vi "sppf single step.vi"(6 "do update":bool, 7 "dt":dbl, 8 "num green photons":dbl, 9 "num red photons":dbl, 10 "w":dbl[][](array[numeric])=[[1e-09, 0.0], [0.0, 1e-09]], 11 "theta":dbl[](array[numeric])=[0.0, 0.0]) -> (1 "wjjm1":dbl[][](array[numeric]), 2 "w":dbl[][](array[numeric]), 3 "theta":dbl[](array[numeric]))   [LabVIEW 2010]
uses:
  <vilib>/Analysis/baseanly.llb/Matrix Type of Inverse Matrix.ctl
  <vilib>/Analysis/Matrix/Datatypes/RealMatrix.ctl
  <vilib>/Analysis/Matrix/Numeric/Multiply/Multiply - R,RM.vi
  <vilib>/Analysis/Matrix/Numeric/Add/Add - RM,RM.vi
  <vilib>/Analysis/baseanly.llb/Real Inverse Matrix.vi
  <vilib>/Analysis/BLAS.llb/dgemv - General Matrix-Vector Product (DBL).vi
  <vilib>/Analysis/Matrix/NI_Matrix.lvlib
  <vilib>/Analysis/NI_AALBase.lvlib
  <vilib>/Analysis/NI_AALBLAS.lvlib
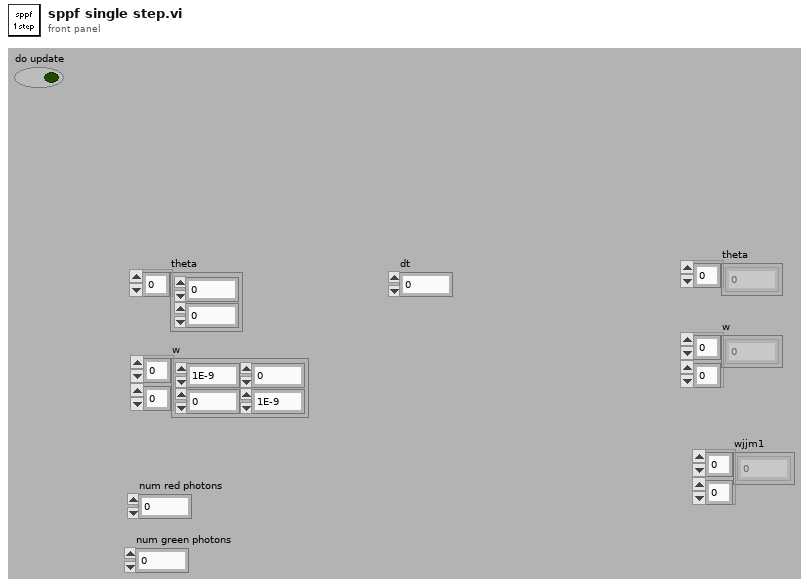
[diagram p1: front panel]
types:
  T1 = typedef "NI_Matrix.lvlib/RealMatrix.ctl" = dbl[][]
  T2 = typedef "NI_AALBase.lvlib/Matrix Type of Inverse Matrix.ctl" = enum32{"General", "Positive Definite", "Lower Triangular", "Upper Triangular"}
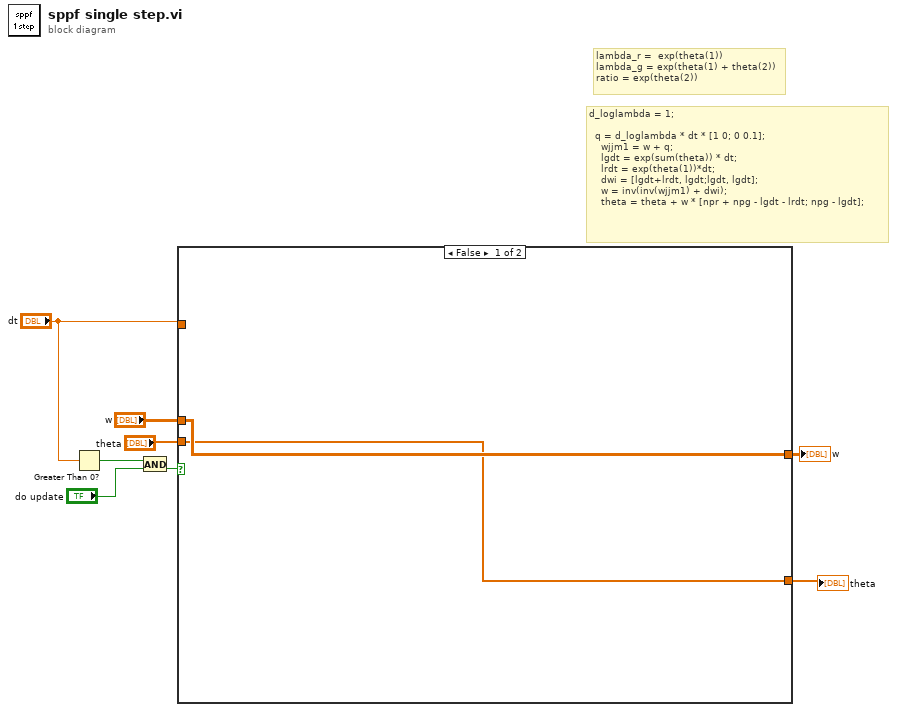
[diagram p0: block diagram]
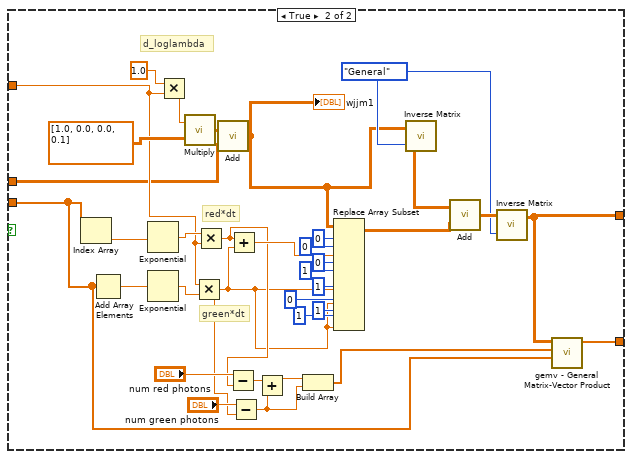
[diagram p2: hidden frame]
diagram:
  # "d_loglambda = 1;\n  \n  q = d_loglambda * dt * [1 0; 0 0.1];\n    wjjm1 = w + q;\n    lgdt = exp(sum(theta)) * dt;\n    lrdt = exp(theta(1))*dt;\n    dwi = [lgdt+lrdt, lgdt;lgdt, lgdt];\n    w = inv(inv(wjjm1) + dwi);\n    theta = theta + w * [npr + npg - lgdt - lrdt; npg - lgdt];"
  # "lambda_r =  exp(theta(1))\nlambda_g = exp(theta(1) + theta(2))\nratio = exp(theta(2))"
  n1 = Greater Than 0?(x="dt") -> (x > 0?=w2:bool)
  n2 = And(x=w2, y="do update") -> (x .and. y?=w3:bool)
  n3 = case shown="False" w3 {
    tunnel: "dt" -> [_ w39]
    tunnel: "theta" -> [w9 w17]
    tunnel: [w10 w16] -> w7
    tunnel: "w" -> [w10 w15]
    tunnel: [w9 w14] -> w5
    frame False {
    }
    frame True {
      w26 = Matrix_Type_of_Inverse_Matrix."General" ("matrix type")
      # "d_loglambda"
      # "green*dt"
      # "red*dt"
      n4 = Index Array(array=w17) -> (element=w43:dbl)  [unwired: 1 in]
      n5 = Add Array Elements(numeric array=w17) -> (sum=w42:dbl)
      n6 = Exponential(1:w43) -> (0:w41:dbl)
      n7 = Exponential(1:w42) -> (0:w40:dbl)
      n8 = Multiply(x=1.0, y=w39) -> (x*y=w13:dbl)
      n9 = call-poly <vilib>:"Multiply.vi"("Real Matrix A"=T1 [[1.0, 0.0], [0.0, 0.1]] ("Real Matrix"), "Real Scalar c"=w13) -> ("c * A"=w44:T1)
      n10 = Multiply(x=w39, y=w40) -> (x*y=w22:dbl)
      n11 = Multiply(x=w41, y=w39) -> (x*y=w24:dbl)
      n12 = call-poly <vilib>:"Add.vi"("Real Matrix B"=w15, "Real Matrix A"=w44) -> ("A + B"=w11:T1)
      "wjjm1" <- w11
      n13 = Subtract(x="num red photons", y=w24) -> (x-y=w21:dbl)
      n14 = Add(x=w24, y=w22) -> (x+y=w30:dbl)
      n15 = Subtract(x="num green photons", y=w22) -> (x-y=w19:dbl)
      n16 = Add(x=w21, y=w19) -> (x+y=w20:dbl)
      n17 = Build Array(w20, w19) -> (w18:dbl[])
      n18 = Replace Array Subset(array=w11, new element #1=w30, index (row) #1=0 ("disabled index (row)"), index (col) #1=0 ("disabled index (col)"), new element #2=w22, index (row) #2=0 ("index (row)"), index (col) #2=1 ("disabled index (col)"), new element #3=w22, index (row) #3=1 ("index (row)"), index (col) #3=0 ("disabled index (col)"), new element #4=w22, index (row) #4=1 ("index (row)"), index (col) #4=1 ("disabled index (col)")) -> (w28:T1)
      n19 = call-poly <vilib>:"Inverse Matrix.vi"("matrix type"=w26, "Input Matrix"=w11) -> ("Inverse Matrix"=w29:T1)  [unwired: 1 out]
      n20 = call-poly <vilib>:"Add.vi"("Real Matrix B"=w28, "Real Matrix A"=w29) -> ("A + B"=w27:T1)
      n21 = call-poly <vilib>:"Inverse Matrix.vi"("matrix type"=w26, "Input Matrix"=w27) -> ("Inverse Matrix"=w16:T1)  [unwired: 1 out]
      n22 = call-poly <vilib>:"gemv - General Matrix-Vector Product.vi"("y"=w17, "x"=w18, "A"=w16) -> ("dgemv"=w14:dbl[])  [unwired: 7 in, 1 out]
    }
  }
  "w" <- w7
  "theta" <- w5
